vi "ManualRenamer.vi"() -> ()   [LabVIEW 2013]
uses:
  <resource>/Framework/Providers/lveio/public/EIOExtName.ctl
panel:
  out "names 2":T1[](array[typedef])
  out "names":T1[](array[typedef])
  out "protocols":string[](array[string])
  in  "Rename":bool
  in  "stop":bool
  in  "NewName":string
  in  "Multicolumn Listbox":i32(listbox)
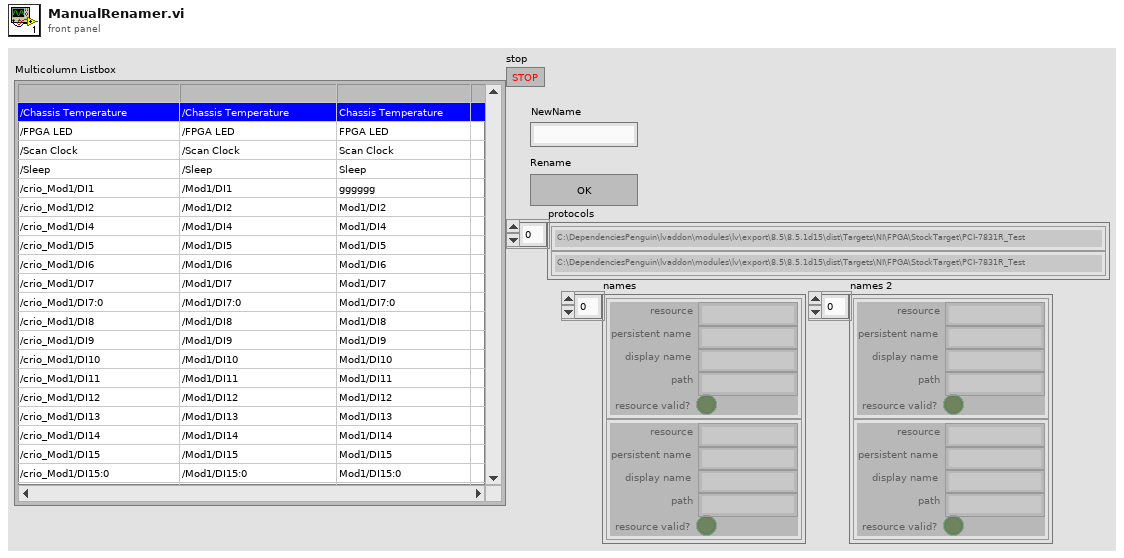
[diagram p1: front panel]
types:
  T1 = typedef "EIOExtName.ctl" = cluster{"resource":string, "persistent name":string, "display name":string, "path":string, "resource valid?":bool}
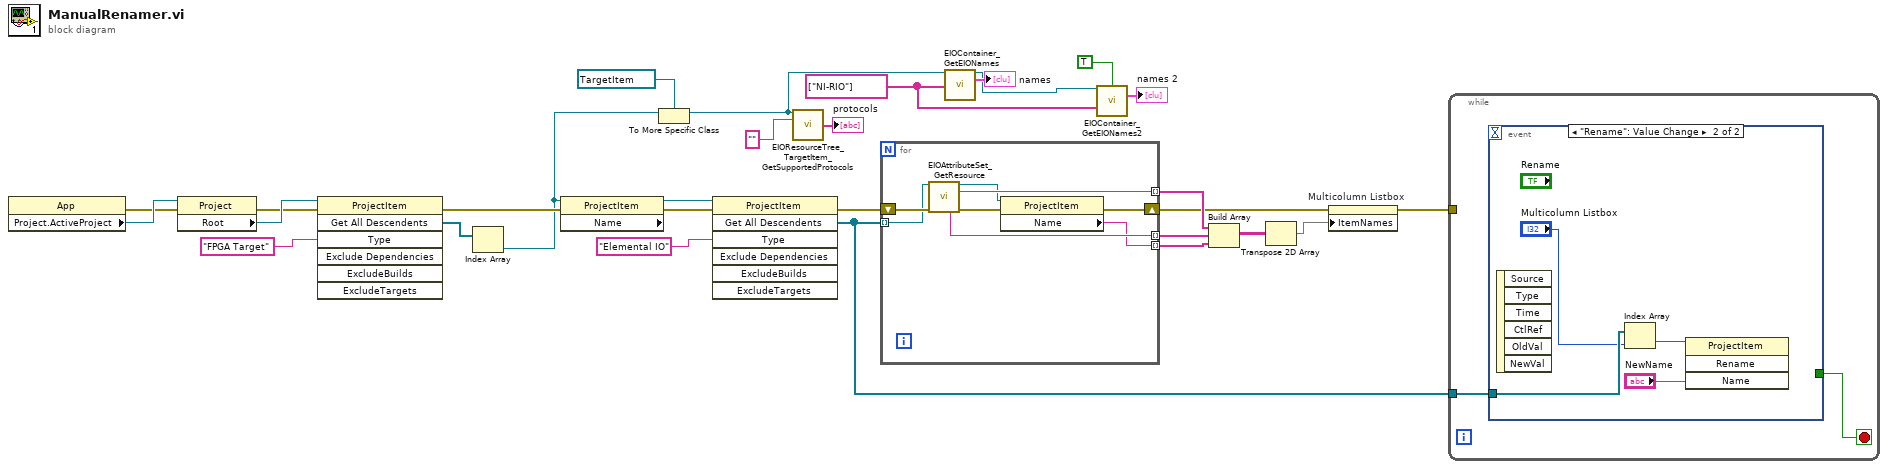
[diagram p0: block diagram]
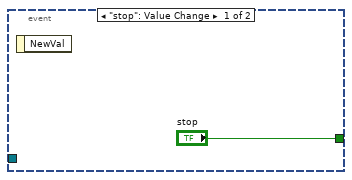
[diagram p2: hidden frame]
diagram:
  w2 = string[] ["NI-RIO"] ("include protocols")
  n1 = property class="App"() -> (error out=w28:errorcluster, "Project.ActiveProject"=w29:refnum<vi>)  [unwired: 2 in, 1 out]
  n2 = property class="Project"(reference=w29, error in=w28) -> (error out=w26:errorcluster, "Root"=w27:refnum<vi>)  [unwired: 1 out]
  n3 = invoke class="ProjectItem" method="Get All Descendents"(reference=w27, error in=w26, "Type"="FPGA Target") -> (error out=w24:errorcluster, "All Descendents"=w13:refnum<vi>[])  [unwired: 4 in, 5 out]
  n4 = Index Array(array=w13) -> (element=w10:refnum<vi>)  [unwired: 1 in]
  n5 = property class="ProjectItem" props=["Name"](reference=w10, error in=w24) -> (reference out=w23:refnum<vi>, error out=w22:errorcluster)  [unwired: 1 out]
  n6 = To More Specific Class(target class=refnum<vi> refnum ("Refnum out"), reference=w10) -> (specific class reference=w6:refnum<vi>)  [unwired: 1 in, 1 out]
  n7 = invoke class="ProjectItem" method="Get All Descendents"(reference=w23, error in=w22, "Type"="Elemental IO") -> (error out=w20:errorcluster, "All Descendents"=w11:refnum<vi>[])  [unwired: 4 in, 5 out]
  n8 = call <resource>:"EIOResourceTree_TargetItem_GetSupportedProtocols.vi"("Refnum In"=w6, "node name"="") -> ("protocols"=→"protocols":string[])  [unwired: 9 in, 4 out]
  n9 = for {
    tunnel: w11 -> [w35] mode=indexing
    shift-right: [w32] -> w15
    shift-left: w20 -> [w37]
    tunnel: [w34] -> w19 mode=indexing
    tunnel: [w33] -> w18 mode=indexing
    tunnel: [w31] -> w14 mode=indexing
    n10 = call <resource>:"EIOAttributeSet_GetResource.vi"("EIOItem Refnum In"=w35, "error in (no error)"=w37) -> ("EIOItem Refnum Out"=w30:refnum<vi>, "resource name"=w34:string, "resource display name"=w33:string, "error out"=w36:errorcluster)  [unwired: 8 in, 2 out]
    n11 = property class="ProjectItem"(reference=w30, error in=w36) -> (error out=w32:errorcluster, "Name"=w31:string)  [unwired: 1 out]
  }
  n12 = call <resource>:"EIOContainer_GetEIONames.vi"("TargetItem Refnum In"=w6, "include protocols"=w2) -> ("TargetItem Refnum Out"=w3:refnum<vi>, "names"=→"names":T1[])  [unwired: 11 in, 1 out]
  n13 = call <resource>:"EIOContainer_GetEIONames2.vi"("TargetItem Refnum In"=w3, "includeHidden"=TRUE, "include protocols"=w2) -> ("names"=→"names 2":T1[])  [unwired: 10 in, 2 out]
  n14 = Build Array(w19, w18, w14) -> (w17:string[][])
  n15 = Transpose 2D Array(2D array=w17) -> (transposed array=w16:string[][])
  n16 = property on="Multicolumn Listbox" class="MCListbox (strict)"(error in=w15, "ItemNames"=w16) -> (error out=w12:errorcluster)  [unwired: 1 in, 1 out]
  n17 = while {
    tunnel: w12 -> [_]
    tunnel: w11 -> [w38]
    stop <- w39 stop-if-true
    n18 = event shown="[1] \"Rename\": Value Change" {
      selector: _ -> [_ _]
      dyn-events: _ -> [_ _]
      timeout: _ -> [_ _]
      tunnel: ["stop" _] -> w39
      tunnel: w38 -> [_ w44]
      event "stop": Value Change {
        n19 = event-data() -> ()  [unwired: 1 in, 1 out]
      }
      event "Rename": Value Change {
        n20 = event-data() -> ()  [unwired: 1 in, 6 out]
        n21 = Index Array(array=w44, index="Multicolumn Listbox") -> (element=w42:refnum<vi>)
        n22 = invoke class="ProjectItem" method="Rename"(reference=w42, "Name"="NewName") -> ()  [unwired: 2 in, 4 out]
      }
    }
  }
